vi "Simultaneous reading of analog and digital signals.vi"() -> ()   [LabVIEW 2023]
uses:
  <vilib>/Utility/error.llb/DialogType.ctl
  <vilib>/DAQmx/read.llb/DAQmx Read (Analog 1D Wfm NChan NSamp).vi
  <vilib>/DAQmx/read.llb/DAQmx Read (Digital 1D Wfm NChan NSamp).vi
  <vilib>/DAQmx/create/channels.llb/DAQmx Create Channel (DI-Digital Input).vi
  <vilib>/DAQmx/configure/timing.llb/DAQmx Timing (Sample Clock).vi
  <vilib>/DAQmx/create/channels.llb/DAQmx Create Channel (CO-Pulse Generation-Time).vi
  <vilib>/DAQmx/create/channels.llb/DAQmx Create Channel (AI-Voltage-Basic).vi
  <vilib>/DAQmx/configure/trigger.llb/DAQmx Start Trigger (Digital Edge).vi
  <vilib>/DAQmx/miscellaneous.llb/DAQmx Fill In Error Info.vi
  <vilib>/Waveform/DWDTOps.llb/DWDT Digital to Binary U8.vi
panel:
  out "Array":string[](array[string])
  in  "Stop Generation":bool caption="Stop Waveform Acquisition"
  out "Digital Waveform Graph":digitalwaveform[](graph)
  out "Waveform Graph":waveform(dbl)[](graph)
  in  "Digital Channels":tag
  in  "Sampling rate (10 x Square Wave Frequency)":dbl=1000.0 format="%0.2f"
  in  "Analog Input Channels":tag
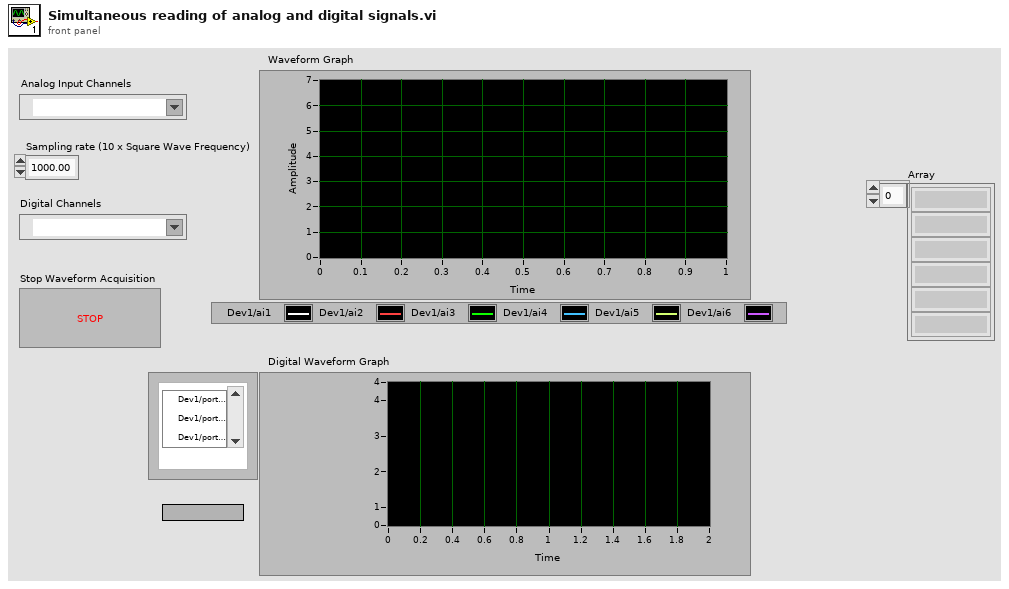
[diagram p1: front panel]
types:
  T1 = enum16{"open", "open or create", "create or replace", "create", "open (read-only)"}
  T2 = typedef "DialogType.ctl" = u16
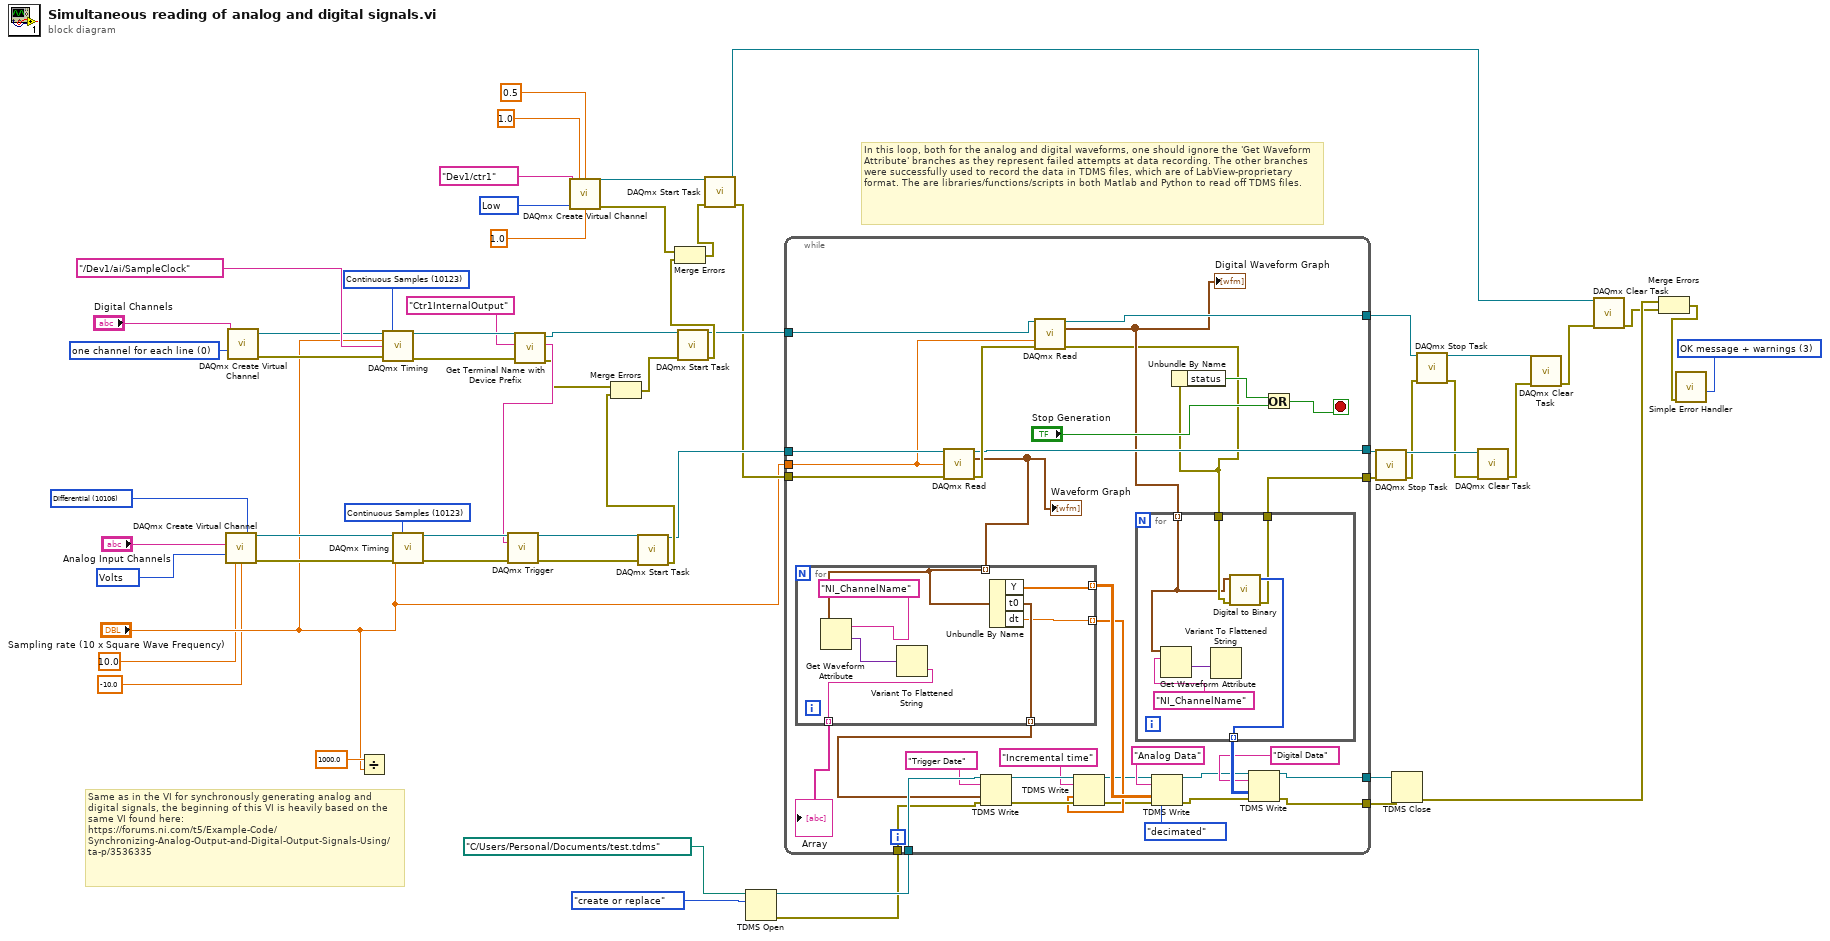
[diagram p0: block diagram]
diagram:
  w24 = T2 3 items=["no dialog", "OK message", "continue or stop message", "OK message + warnings", "continue/stop + warnings"] ("type of dialog (OK msg:1)")
  w38 = 10214 items=["High"=10192, "Low"=10214] ("idle state")
  w48 = 10123 items=["Finite Samples"=10178, "Continuous Samples"=10123, "Hardware Timed Single Point"=12522] ("sample mode")
  w51 = 0 items=["one channel for each line", "one channel for all lines"] ("line grouping")
  w56 = 10123 items=["Finite Samples"=10178, "Continuous Samples"=10123, "Hardware Timed Single Point"=12522] ("sample mode")
  w14 = 10348 items=["Volts"=10348, "From Custom Scale"=10065] ("units")
  w59 = 10106 items=["Default"=-1, "RSE"=10083, "NRSE"=10078, "Differential"=10106, "Pseudodifferential"=12529] ("input terminal configuration")
  # "In this loop, both for the analog and digital waveforms, one should ignore the 'Get Waveform Attribute' branches as they represent failed attempts at data recording. The other branches were successfully used to record the data in TDMS files, which are of LabView-proprietary format. The are libraries/functions/scripts in both Matlab and Python to read off TDMS files."
  # "Same as in the VI for synchronously generating analog and digital signals, the beginning of this VI is heavily based on the same VI found here:\nhttps://forums.ni.com/t5/Example-Code/Synchronizing-Analog-Output-and-Digital-Output-Signals-Using/ta-p/3536335"
  n1 = call-poly <vilib>:"DAQmx Create Virtual Channel.vi"("maximum value"=10.0, "minimum value"=-10.0, "input terminal configuration"=w59, "physical channels"="Analog Input Channels", "units"=w14) -> ("task out"=w58:refnum<k21>, "error out"=w57:errorcluster)  [unwired: 9 in]
  n2 = call-poly <vilib>:"DAQmx Create Virtual Channel.vi"("lines"="Digital Channels", "line grouping"=w51) -> ("task out"=w47:refnum<k21>, "error out"=w46:errorcluster)  [unwired: 12 in]
  n3 = Divide(x=1000.0, y="Sampling rate (10 x Square Wave Frequency)") -> ()  [unwired: 1 out]
  n4 = call-poly <vilib>:"DAQmx Timing.vi"("task/channels in"=w47, "sample mode"=w48, "rate"="Sampling rate (10 x Square Wave Frequency)", "source"=tag "/Dev1/ai/SampleClock", "error in"=w46) -> ("task out"=w45:refnum<k21>, "error out"=w44:errorcluster)  [unwired: 9 in]
  n5 = call-poly <vilib>:"DAQmx Timing.vi"("task/channels in"=w58, "sample mode"=w56, "rate"="Sampling rate (10 x Square Wave Frequency)", "error in"=w57) -> ("task out"=w55:refnum<k21>, "error out"=w54:errorcluster)  [unwired: 10 in]
  n6 = call "Get Terminal Name with Device Prefix.vi"("error in (no error)"=w44, "Local Terminal Name"="Ctr1InternalOutput", "task/channels in"=w45) -> ("error out"=w41:errorcluster, "Terminal Name with Device Prefix"=w43:tag, "task out"=w39:refnum<k21>)  [unwired: 6 in]
  n7 = call-poly <vilib>:"DAQmx Trigger.vi"("task/channels in"=w55, "source"=w43, "error in"=w54) -> ("task out"=w53:refnum<k21>, "error out"=w52:errorcluster)  [unwired: 11 in]
  n8 = call-poly <vilib>:"DAQmx Create Virtual Channel.vi"("high time"=1.0, "low time"=0.5, "counter"=tag "Dev1/ctr1", "idle state"=w38, "initial delay"=1.0) -> ("task out"=w29:refnum<k21>, "error out"=w31:errorcluster)  [unwired: 9 in]
  n9 = call <vilib>:"DAQmx Start Task.vi"("task/channels in"=w53, "error in"=w52) -> ("task out"=w28:refnum<k21>, "error out"=w42:errorcluster)  [unwired: 12 in]
  n10 = Merge Errors(w41, w42) -> (w40:errorcluster)
  n11 = call <vilib>:"DAQmx Start Task.vi"("task/channels in"=w39, "error in"=w40) -> ("task out"=w27:refnum<k21>, "error out"=w32:errorcluster)  [unwired: 12 in]
  n12 = Merge Errors(w31, w32) -> (w30:errorcluster)
  n13 = call <vilib>:"DAQmx Start Task.vi"("task/channels in"=w29, "error in"=w30) -> ("task out"=w17:refnum<k21>, "error out"=w26:errorcluster)  [unwired: 12 in]
  n14 = TDMS Open(10:T1."create or replace" ("operation (0:open)"), 11:path "C:/Users/Personal/Documents/test.tdms" ("Save Data To:")) -> (0:w9:errorcluster, 3:w10:refnum<k34>)  [unwired: 5 in]
  n15 = while {
    tunnel: w28 -> [w94]
    tunnel: w27 -> [w93]
    tunnel: w26 -> [w92]
    tunnel: [w90] -> w25
    tunnel: [w86] -> w21
    tunnel: "Sampling rate (10 x Square Wave Frequency)" -> [w84]
    tunnel: w10 -> [w81]
    tunnel: w9 -> [w80]
    tunnel: [w64] -> w8
    tunnel: [w65] -> w7
    tunnel: [w63] -> w3
    stop <- w87 stop-if-true
    n16 = call-poly <vilib>:"DAQmx Read.vi"("task/channels in"=w94, "number of samples per channel"=w84, "error in"=w92) -> ("task out"=w90:refnum<k21>, "data"=w83:waveform(dbl)[], "error out"=w91:errorcluster)  [unwired: 10 in]
    "Waveform Graph" <- w83
    n17 = for {
      tunnel: w83 -> [w104] mode=indexing
      tunnel: [w107] -> w82 mode=indexing
      tunnel: [w106] -> w78 mode=indexing
      tunnel: [w105] -> w74 mode=indexing
      tunnel: [w101] -> w61 mode=indexing
      n18 = Get Waveform Attribute(6:"NI_ChannelName" ("name"), 7:w104) -> (1:w102:variant)  [unwired: 2 in, 3 out]
      n19 = Variant To Flattened String(Variant=w102) -> (data string=w101:string)  [unwired: 1 out]
      n20 = Unbundle By Name(w104) -> ("Y"=w107:dbl[], "t0"=w106:timestamp, "dt"=w105:dbl)
    }
    "Array" <- w61
    n21 = TDMS Write(0:w81, 5:"Trigger Date" ("group name in (Untitled)"), 9:w78, 11:w80) -> (4:w77:refnum<k34>, 15:w76:errorcluster)  [unwired: 2 in, 2 out]
    n22 = call-poly <vilib>:"DAQmx Read.vi"("task/channels in"=w93, "timeout"=w84, "error in"=w91) -> ("task out"=w86:refnum<k21>, "data"=w71:digitalwaveform[], "error out"=w66:errorcluster)  [unwired: 10 in]
    "Digital Waveform Graph" <- w71
    n23 = TDMS Write(0:w77, 5:"Incremental time" ("group name in (Untitled)"), 9:w74, 11:w76) -> (4:w73:refnum<k34>, 15:w72:errorcluster)  [unwired: 2 in, 2 out]
    n24 = for {
      tunnel: w71 -> [w97] mode=indexing
      tunnel: [w100] -> w70 mode=indexing
      tunnel: w66 -> [w99]
      tunnel: [w98] -> w63
      n25 = Get Waveform Attribute(6:"NI_ChannelName" ("name"), 7:w97) -> (1:w95:variant)  [unwired: 2 in, 3 out]
      n26 = Variant To Flattened String(Variant=w95) -> ()  [unwired: 2 out]
      n27 = call-poly <vilib>:"Digital to Binary.vi"("error in (no error)"=w99, "digital waveform"=w97) -> ("error out"=w98:errorcluster, "binary array"=w100:u8[])  [unwired: 8 in]
    }
    n28 = TDMS Write(0:w73, 1:enum16{"decimated", "interleaved"}."decimated" ("data layout (0:decimated)"), 5:"Analog Data" ("group name in (Untitled)"), 9:w82, 11:w72) -> (4:w68:refnum<k34>, 15:w67:errorcluster)  [unwired: 1 in, 2 out]
    n29 = Unbundle By Name(w66) -> ("status"=w89:bool)
    n30 = TDMS Write(0:w68, 5:"Digital Data" ("group name in (Untitled)"), 9:w70, 11:w67) -> (4:w65:refnum<k34>, 15:w64:errorcluster)  [unwired: 2 in, 2 out]
    n31 = Or(x=w89, y="Stop Generation") -> (x .or. y?=w87:bool)
  }
  n32 = call <vilib>:"DAQmx Stop Task.vi"("task/channels in"=w25, "error in"=w3) -> ("task out"=w23:refnum<k21>, "error out"=w22:errorcluster)  [unwired: 12 in]
  n33 = TDMS Close(8:w8, 11:w7) -> (0:w6:errorcluster)  [unwired: 1 out]
  n34 = call <vilib>:"DAQmx Stop Task.vi"("task/channels in"=w21, "error in"=w22) -> ("task out"=w20:refnum<k21>, "error out"=w19:errorcluster)  [unwired: 12 in]
  n35 = call <vilib>:"DAQmx Clear Task.vi"("task in"=w23, "error in"=w19) -> ("error out"=w18:errorcluster)  [unwired: 13 in]
  n36 = call <vilib>:"DAQmx Clear Task.vi"("task in"=w20, "error in"=w18) -> ("error out"=w16:errorcluster)  [unwired: 13 in]
  n37 = call <vilib>:"DAQmx Clear Task.vi"("task in"=w17, "error in"=w16) -> ("error out"=w5:errorcluster)  [unwired: 13 in]
  n38 = Merge Errors(w6, w5) -> (w4:errorcluster)
  n39 = call <vilib>:"Simple Error Handler.vi"("type of dialog (OK msg:1)"=w24, "error in (no error)"=w4) -> ()  [unwired: 3 in, 5 out]
